vi "Topo & GridSpectr_DriftCorrection_zSpec_v19.vi"(6 "Internal use":string, 7 "Grid param":T1 {"height (m)" format="%#_6p"; "width (m)" format="%#_6p"; "center Y (m)" format="%#_6p"; "center X (m)" format="%#_6p"}, 8 "Error in (no error)":errorcluster, 9 "Points Y/Index Y":i32, 10 "Points X/Index X":i32, 11 "Method":enum16{"init", "run", "end"}(ring)=enum."end") -> (0 "Error out":errorcluster)   [LabVIEW 2014]
doc: "Example of a measurement VI to be used in the \"Experiments on a Grid\" tool as external VI.\n\nThis example measure the topography and spectroscopy data. The spectroscopy measurements are taken on a subgrid. The data are saved to a sxm and a binary file.\n\n- Nanonis Programming Interface -"
uses:
  <userlib>/Nanonis Prog Interface V5/Scan/Grid/GridPatternGet.vi
  <userlib>/Nanonis Prog Interface V5/Scan/Grid/LinePatternGet.vi
  <userlib>/Nanonis Prog Interface V5/Nanonis Prog Interface.lvlib
panel:
  in  "PLL ON/OFF":bool=TRUE
  in  "Spectroscopy":u16(ring) items=["Bias", "zSpec"]
  in  "autoStop":bool
  in  "trigger 2 >Hz":sgl format="%#_6p"
  in  "trigger1 < Hz":sgl format="%#_6p"
  out "zFile":refnum<file>
  out "last z adjustment":sgl=-8.2707174e-12 format="%#_6p"
  in  "during Spec Bias (V)":sgl=-0.1 format="%#_5p"
  in  "type":u16(ring)=1 items=["Line", "Grid"]
  in  "readjust setpoint every":i32=1
  in  "Correct Drift":bool=TRUE
  in  "Email when finished":string="cornelius.krull@monash.edu,Dhaneesh.Gopalakrishnan@monash.edu,marina.castelli@monash.edu"
  in  "STS z offset":dbl=2e-10 format="%#_6p"
  out "ETA":timestamp=timestamp(3575267058.899443 s since 1904-01-01)
  out "remaining":dbl format="%<%H:%M:%S>t"
  out "Progress":u8(slide)=100 scale=0.0..100.0 scale format="%#.1g"
  out "total Points":i32=2500
  in  "preSTS delay [ms]":u32=500
  in  "ref Bias":dbl=-0.1 format="%#_6p"
  in  "Imaging Bias":dbl=0.02 format="%#_6p"
  in  "max applied Drift Correction":i32=20 min=1 max=100 step=1 format="%.0p"
  in  "Correlate":u16(ring) items=["first Frame", "successive Frames"]
  out "Topo Images taken":i32=50
  in  "Increment":i32=8
  in  "Threshold":i32=2 min=1 step=1
  in  "tip Speed (m/s)":sgl=2e-09 format="%.2p"
  out "X drift":i32=1
  out "Y drift":i32
  out "Last Drift detected":i32=1
  in  "MaxImagesBack":i32=2
  in  "Channel index (0-23)":u8(ring) items=["Current"=0, "Z (m)"=14]
  in  "File name":string="symmetric_node_zOff=200p"
  in  "ref Current":dbl=7e-11 format="%#_6p"
  in  "Imaging Current":dbl=1e-11 format="%#_6p"
  in  "zdrift \nDuration (s)":dbl
  in  "Correct z drift":bool
  out "Status":string="finishing"
  in  "Drift correction Pixels":i32=256 caption="Topo Pixels"
  out "Y Offset":dbl=-4.101562475072873e-10 format="%#_6p"
  out "X Offset":dbl=4.687499971511855e-10 format="%#_6p"
  out "Points taken":dbl=2500.0
  in  "Drift Correction every":i32=80
  # "z Spectroscopy"
  # "GRID points"
  # "Increase this if no Drift was detected for \na certain number of images"
  # "%"
  # "time (HH:MM:SS)"
  # "images back"
  # "% of image size"
  # "RUN smart tilt before starting the GRID\nImg Angle = 0  CHECK CUTOFF\nmove tip to reference point for tip height"
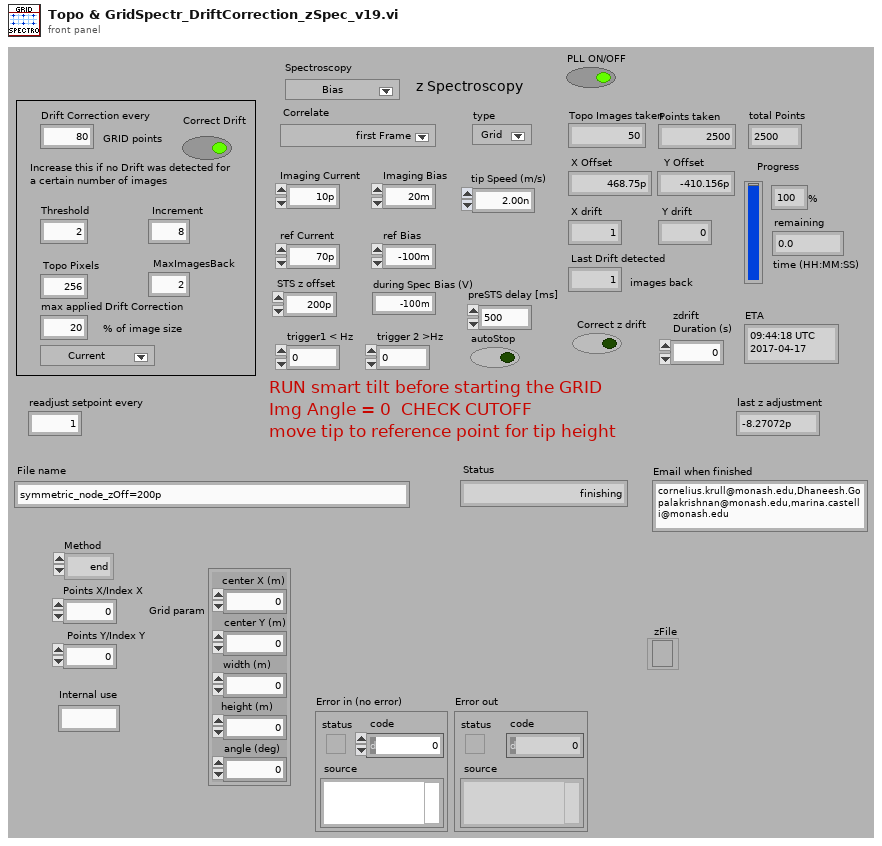
[diagram p1: front panel]
types:
  T1 = cluster{"center X (m)":sgl, "center Y (m)":sgl, "width (m)":sgl, "height (m)":sgl, "angle (deg)":sgl}
  T2 = enum16{"open", "replace", "create", "open or create", "replace or create", "replace or create with confirmation"}
  T3 = cluster{"Drift correction Pixels":i32, "Imaging Current":dbl, "STS Current":dbl, "MaxImagesBack":i32, "tip Speed (m/s)":sgl, "Threshold":i32, "Increment":i32, "Correlate":u16, "max applied Drift Correction":i32, "Imaging Bias":dbl, "Move Current":dbl, "Move Bias":dbl, "STS Bias":dbl, "preSTS delay [ms]":u32, "STS z offset":dbl, "Correct Drift":bool, "Lockin ON/OFF":bool}
  T4 = cluster{"x(m)":sgl, "y(m)":sgl, "Text":string, "Color":u32}
  T5 = cluster{"Z averaging time (s)":sgl, "Z offset (m)":sgl, "Initial settling time (s)":sgl}
  T6 = cluster{"center X":sgl, "center Y":sgl, "angle":sgl, "width":sgl, "height":sgl, "# pixels":i32, "# lines":i32}
  T7 = cluster{"Name":string, "Calibration":sgl, "Offset":sgl, "Channel index":i32}[]
  T8 = cluster{"up/down":bool, "time/line":sgl, "start time":timestamp, "end time":timestamp}
  T9 = cluster{"X (m)":sgl, "Y (m)":sgl, "Text":string, "Color":u32, "Visible":bool}[]
  T10 = cluster{"Max. slew rate (V/s)":sgl, "Settling time (s)":sgl, "Integration time (s)":sgl}
  T11 = cluster{"End settling time (s)":sgl, "Z control time (s)":sgl}
  T12 = cluster{"Z averaging time (s)":sgl, "Initial settling time (s)":sgl}
  T13 = cluster{"Max. slew rate (m/s)":sgl, "Settling time (s)":sgl, "Integration time (s)":sgl}
  T14 = cluster{"Points X/Index X":i32, "Points Y/Index Y":i32}
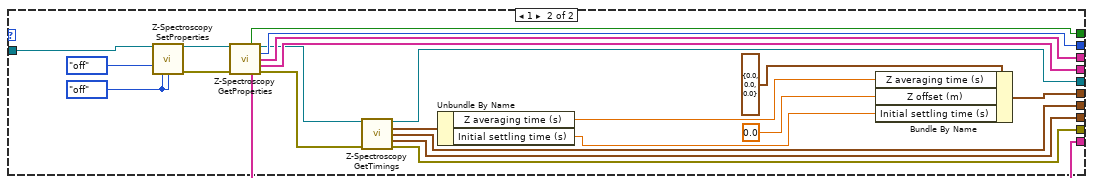
[diagram p3: hidden frame]
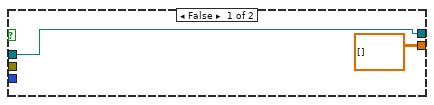
[diagram p4: hidden frame]
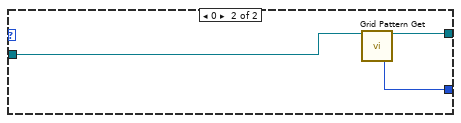
[diagram p5: hidden frame]
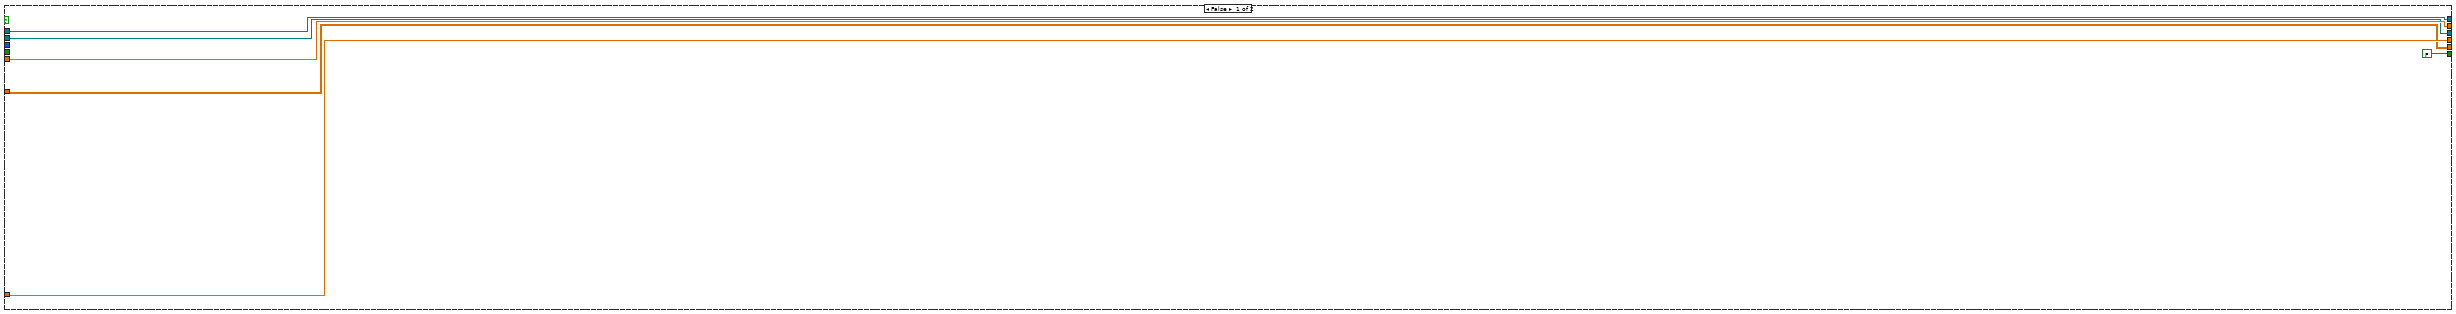
[diagram p10: hidden frame]
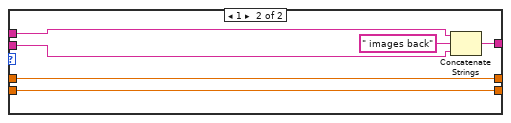
[diagram p11: hidden frame]
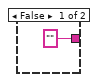
[diagram p13: hidden frame]
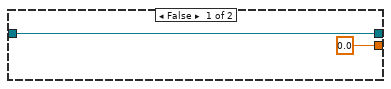
[diagram p14: hidden frame]
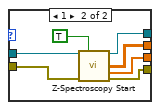
[diagram p16: hidden frame]
diagram:
  n1 = while {
    shift-right: [w21] -> _
    shift-left: _ -> [w38]
    shift-right: [w33] -> _
    shift-left: _ -> [w32]
    shift-right: [w30] -> _
    shift-left: _ -> [w31]
    shift-right: [w29] -> _
    shift-left: _ -> [w28]
    shift-right: [w27] -> _
    shift-left: _ -> [w26]
    shift-right: [w25] -> _
    shift-left: _ -> [w24]
    shift-right: [w23] -> _
    shift-left: _ -> [w22]
    shift-right: [w20] -> _
    shift-left: _ -> [w19]
    shift-right: [w18] -> _
    shift-left: _ -> [w17]
    shift-right: [w16] -> _
    shift-left: _ -> [w9]
    shift-right: [w15] -> _
    shift-left: _ -> [w8]
    shift-right: [w14] -> _
    shift-left: _ -> [w11]
    shift-right: [w13] -> _
    shift-left: _ -> [w10]
    shift-right: [w6] -> _
    shift-left: _ -> [w5]
    stop <- TRUE stop-if-true
    n2 = case shown="\"run\"" "Method" {
      tunnel: [w63 w296 _] -> w21
      tunnel: w38 -> [_ w296 w533]
      tunnel: "Error in (no error)" -> [w136 w289 w561]
      tunnel: [w118 w295 w501] -> w36
      tunnel: "Points X/Index X" -> [w56 w290 _]
      tunnel: "Points Y/Index Y" -> [w55 w283 _]
      tunnel: [w162 w293 w550] -> w33
      tunnel: w32 -> [_ w294 w550]
      tunnel: w31 -> [_ w292 w543]
      tunnel: [w154 w291 _] -> w30
      tunnel: [w152 w233 w573] -> w29
      tunnel: w28 -> [_ w233 w573]
      tunnel: [w108 w276 w512] -> w27
      tunnel: w26 -> [_ w260 w537]
      tunnel: ["Grid param" w286 _] -> w25
      tunnel: w24 -> [_ w286 w560]
      tunnel: [w134 w251 _] -> w23
      tunnel: w22 -> [_ w251 w568]
      tunnel: [w55 w284 w551] -> w20
      tunnel: w19 -> [_ w284 w551]
      tunnel: [w56 w285 w552] -> w18
      tunnel: w17 -> [_ w285 w552]
      tunnel: [w145 w266 w549] -> w16
      tunnel: [w145 w271 w547] -> w15
      tunnel: [w130 w265 w544] -> w14
      tunnel: [0 w249 w548] -> w13
      tunnel: w10 -> [_ w235 w548]
      tunnel: "Drift Correction every" -> [_ w279 _]
      tunnel: w11 -> [_ w270 w544]
      tunnel: w9 -> [_ w277 w549]
      tunnel: w8 -> [_ w263 w547]
      tunnel: "Drift correction Pixels" -> [w129 _ _]
      tunnel: [w105 w268 _] -> w6
      tunnel: w5 -> [_ w269 w545]
      tunnel: "Correct z drift" -> [_ w267 _]
      tunnel: "Channel index (0-23)" -> [w87 w264 _]
      tunnel: "MaxImagesBack" -> [w128 _ _]
      tunnel: "Correlate" -> [w114 _ _]
      frame "init", Default {
        w65 = 0.0 ("Move Current")
        w145 = 0.0
        # "- Get bias spectroscopy parameters\n- Open binary file for spectr. data"
        # "initialize Z buffer"
        # "Get index of Z in Signal list"
        n3 = case shown="0, Default" w114 {
          frame 0, Default {
            n4 = local write "MaxImagesBack"(2 ("StepsBack")) -> ()
          }
          frame 1 {
          }
        }
        n5 = call <userlib>:"Prog Interface - OpenAppRef.vi"("Error in (no error)"=w136) -> ("Error out"=w83:errorcluster, "Application reference"=w84:refnum<vi>)  [unwired: 5 in]
        n6 = local write "Status"("init" ("Status")) -> ()
        n7 = call <userlib>:"XY-Pos Get.vi"("error in (no error)"=w83, "Application ref in"=w84) -> ("error out"=w52:errorcluster, "Y (m)"=w77:sgl, "X (m)"=w78:sgl, "Application ref out"=w48:refnum<vi>)  [unwired: 5 in]
        n8 = call <userlib>:"Points Get.vi"("Application ref in"=w48) -> ("Application ref out"=w47:refnum<vi>, "Points"=w49:T9)  [unwired: 12 in, 1 out]
        n9 = for {
          tunnel: w49 -> [w169] mode=indexing
          tunnel: [w163] -> w44 mode=indexing
          n10 = Unbundle By Name(w169) -> ("X (m)"=w167:sgl, "Y (m)"=w166:sgl, "Text"=w165:string, "Color"=w164:u32)  [unwired: 1 out]
          n11 = Bundle By Name(cluster=T4 {"x(m)"=0.0, "y(m)"=0.0, "Text"="", "Color"=16777216} ("Point"), "x(m)"=w167, "y(m)"=w166, "Text"=w165, "Color"=w164) -> (w163:T4)
        }
        n12 = Bundle By Name(cluster=cluster{"X (m)":sgl, "Y (m)":sgl} {"X (m)"=0.0, "Y (m)"=0.0} ("Point Coordinates"), "X (m)"=w78, "Y (m)"=w77) -> (w79:cluster{"X (m)":sgl, "Y (m)":sgl})
        n13 = call <userlib>:"Point Erase.vi"("Application ref in"=w47, "Point index (-1=All points)"=-1) -> ("Application ref out"=w70:refnum<vi>)  [unwired: 12 in, 1 out]
        n14 = call <userlib>:"Point Draw.vi"("Application ref in"=w70, "Point Coordinates"=w79, "Text"="ref X ref", "Color"=u32 6618880) -> ("Application ref out"=w46:refnum<vi>)  [unwired: 10 in, 1 out]
        n15 = call <userlib>:"Points Draw.vi"("Application ref in"=w46, "Points Configuration"=w44) -> ("Application ref out"=w45:refnum<vi>)  [unwired: 12 in, 1 out]
        n16 = call <userlib>:"Point ShowHide.vi"("Application ref in"=w45, "Point index (-1=All points)"=-1, "Show/Hide"=enum16{"Show", "Hide"}."Show") -> ("Application ref out"=w73:refnum<vi>)  [unwired: 11 in, 1 out]
        n17 = case shown="1, Default" "type" {
          tunnel: [w223 w226] -> w51
          tunnel: [w220 w224] -> w109
          tunnel: w73 -> [w219 w225]
          frame 1, Default {
            n18 = call-poly <userlib>:"Grid Pattern Get.vi"("Application ref in"=w219) -> ("Points Y"=w221:i32, "Points X"=w222:i32, "Application ref out"=w223:refnum<vi>)  [unwired: 10 in, 6 out]
            n19 = Multiply(x=w221, y=w222) -> (x*y=w220:i32)
          }
          frame 0 {
            n20 = call-poly <userlib>:"Grid Pattern Get.vi"("Application ref in"=w225) -> ("Points"=w224:i32, "Application ref out"=w226:refnum<vi>)  [unwired: 12 in, 5 out]
          }
        }
        "total Points" <- w109
        n21 = local write "Topo Images taken"(0 ("Images taken")) -> ()
        n22 = local write "Last Drift detected"(0 ("Last Drift detected")) -> ()
        n23 = call <userlib>:"Get Session Path.vi"("error in (no error)"=w52, "Application ref in"=w51) -> ("error out"=w135:errorcluster, "Session path"=w122:path, "Application ref out"=w116:refnum<vi>)  [unwired: 7 in]
        n24 = local read "Spectroscopy"() -> (w53:u16)
        n25 = Get Date/Time In Seconds() -> (seconds since 1Jan1904=w134:timestamp)
        n26 = case shown="0, Default" w53 {
          tunnel: [w171 w206] -> w158
          tunnel: [w174 w205] -> w156
          tunnel: [w178 w192] -> w155
          tunnel: [w173 w204] -> w151
          tunnel: [w172 w203] -> w149
          tunnel: [w175 w202] -> w148
          tunnel: w116 -> [w180 w195]
          tunnel: [w177 w200] -> w76
          tunnel: [w176 w199] -> w75
          tunnel: [w170 w185] -> w50
          tunnel: [w179 w198] -> w54
          frame 0, Default {
            n27 = call <userlib>:"BiasSpectroscopy SetProperties.vi"("Application ref in"=w180) -> ("Application ref out"=w184:refnum<vi>, "Error out"=w183:errorcluster)  [unwired: 13 in]
            n28 = call <userlib>:"BiasSpectroscopy GetProperties.vi"("Application ref in"=w184, "Error in (no error)"=w183) -> ("Backward sweep"=w171:bool, "Application ref out"=w182:refnum<vi>, "Number of points"=w172:i32, "Channels"=w175:string[], "Parameters"=w174:string[], "Fixed parameters"=w173:string[], "Error out"=w181:errorcluster)  [unwired: 5 in, 2 out]
            n29 = call <userlib>:"BiasSpectroscopy GetTimings.vi"("Application ref in"=w182, "Error in (no error)"=w181) -> ("Application ref out"=w179:refnum<vi>, "Initialization"=w170:T5, "Sweep Timing"=w176:T10, "End of Sweep"=w177:T11, "Error out"=w178:errorcluster)  [unwired: 9 in]
          }
          frame 1 {
            w197 = enum16{"no change", "on", "off"}."off" ("Save dialog")
            n30 = call <userlib>:"Z-Spectroscopy SetProperties.vi"("Application ref in"=w195, "Autosave"=enum16{"no change", "on", "off"}."off" ("Autosave (no change)"), "Save dialog"=w197, "Save all sweeps (no change)"=w197) -> ("Application ref out"=w194:refnum<vi>, "error out"=w193:errorcluster)  [unwired: 10 in]
            n31 = call <userlib>:"Z-Spectroscopy GetProperties.vi"("Application ref in"=w194, "error in (no error)"=w193) -> ("Backward sweep"=w206:bool, "Application ref out"=w201:refnum<vi>, "Number of points"=w203:i32, "Channels"=w202:string[], "Parameters"=w205:string[], "Fixed parameters"=w204:string[], "error out"=w191:errorcluster)  [unwired: 6 in, 1 out]
            n32 = call <userlib>:"Z-Spectroscopy GetTimings.vi"("Application ref in"=w201, "Error in (no error)"=w191) -> ("Application ref out"=w198:refnum<vi>, "Initialization"=w186:T12, "Sweep Timing"=w199:T13, "End of Sweep"=w200:T11, "Error out"=w192:errorcluster)  [unwired: 9 in]
            n33 = Unbundle By Name(w186) -> ("Z averaging time (s)"=w188:sgl, "Initial settling time (s)"=w189:sgl)
            n34 = Bundle By Name(cluster=T5 {"Z averaging time (s)"=0.0, "Z offset (m)"=0.0, "Initial settling time (s)"=0.0} ("Initialization"), "Z averaging time (s)"=w188, "Z offset (m)"=sgl 0.0, "Initial settling time (s)"=w189) -> (w185:T5)
          }
        }
        n35 = call "Create Filenames (SubVI).vi"("error in (no error)"=w135, "seconds since 1Jan1904"=w134, "File name"="File name", "Session path"=w122) -> ("error out"=w125:errorcluster, "binFilePath"=w119:path, "topoFilePath"=w63:path, "Drift File out"=w106:refnum<file>)  [unwired: 4 in]
        n36 = Strip Path(path=w63) -> (stripped path=w62:path)  [unwired: 1 out]
        n37 = Strip Path(path=w119) -> (stripped path=w121:path)  [unwired: 1 out]
        n38 = Build Path(base path=w121, name or relative path="topo") -> (appended path=w43:path)
        n39 = Build Path(base path=w62, name or relative path="zAdjustments.txt") -> (appended path=w60:path)
        n40 = Open/Create/Replace File(file path (use dialog)=w60, operation (0:open)=T2."open or create", access (0:read/write)=enum16{"read/write", "read-only", "write-only"}."write-only") -> (refnum out=→"zFile":refnum<file>)  [unwired: 3 in, 2 out]
        n41 = local read "max applied Drift Correction"() -> (w93:i32)
        n42 = local read "Drift correction Pixels"() -> (w101:i32)
        n43 = local read "preSTS delay [ms]"() -> (w90:u32)
        n44 = local read "Imaging Current"() -> (w100:dbl)
        n45 = local read "MaxImagesBack"() -> (w97:i32)
        n46 = local read "tip Speed (m/s)"() -> (w98:sgl)
        n47 = local read "Imaging Bias"() -> (w92:dbl)
        n48 = local read "Correct Drift"() -> (w88:bool)
        n49 = local read "STS z offset"() -> (w89:dbl)
        n50 = local read "ref Current"() -> (w99:dbl)
        n51 = local read "Increment"() -> (w95:i32)
        n52 = local read "Threshold"() -> (w96:i32)
        n53 = local read "Correlate"() -> (w94:u16)
        n54 = local read "ref Bias"() -> (w91:dbl)
        n55 = Bundle By Name(cluster=T3 {"Drift correction Pixels"=256, "Imaging Current"=5e-11, "STS Current"=1e-10, "MaxImagesBack"=2, "tip Speed (m/s)"=1e-08, "Threshold"=2, "Increment"=64, "Correlate"=0, "max applied Drift Correction"=20, "Imaging Bias"=-0.02, "Move Current"=1.5e-11, "Move Bias"=-0.02, "STS Bias"=0.1, "preSTS delay [ms]"=1000, "STS z offset"=-1.7e-10, "Correct Drift"=TRUE, "Lockin ON/OFF"=TRUE} ("Drift Correction"), "Drift correction Pixels"=w101, "Imaging Current"=w100, "STS Current"=w99, "MaxImagesBack"=w97, "tip Speed (m/s)"=w98, "Threshold"=w96, "Increment"=w95, "Correlate"=w94, "max applied Drift Correction"=w93, "Imaging Bias"=w92, "Move Current"=w65, "Move Bias"=w65, "STS Bias"=w91, "preSTS delay [ms]"=w90, "STS z offset"=w89, "Correct Drift"=w88, "Lockin ON/OFF"=FALSE) -> (w103:T3)
        n56 = Bundle("Points X/Index X"=w56, "Points Y/Index Y"=w55) -> (w157:T14)  [unwired: 1 in]
        n57 = call "DriftFileHeader(SubVI).vi"("Byte Stream File in"=w106, "Drift Correction"=w103, "End of Sweep"=w76, "Application ref in"=w54, "Sweep Timing"=w75, "Initialization"=w50) -> ("Byte Stream File out"=w105:refnum<file>, "Application ref out"=w104:refnum<vi>)  [unwired: 8 in]
        n58 = call <userlib>:"Create Header for BinaryFile.vi"("Grid points"=w157, "Grid param"="Grid param", "Fixed parameters"=w151, "Backward sweep"=w158, "Sweep signal"="Bias (V)" ("Sweep Signal"), "Parameters"=w156, "Channels"=w148, "Points per sweep"=w149) -> ("Header (fixed attributes)"=w160:string[][])  [unwired: 3 in]
        n59 = call <userlib>:"Write Header to BinaryFile [ with Save dialog].vi"("Fixed Attributes"=w160, "Show Dialog? (T)"=FALSE, "Filename"=w119) -> ("Error out"=w126:errorcluster, "File ref"=w154:refnum<file>)  [unwired: 5 in, 2 out]
        n60 = local read "Imaging Bias"() -> (w111:dbl)
        n61 = Merge Errors(w126, w125) -> (w127:errorcluster)
        n62 = call "SafeBiasSet.vi"("Application ref in"=w104, "Bias (V)"=w111) -> ("Application ref out"=w42:refnum<vi>)  [unwired: 7 in, 1 out]
        n63 = Merge Errors(w155, w127) -> (w118:errorcluster)
        n64 = call <userlib>:"Set Session Path.vi"("error in (no error)"=w118, "Session Folder"=w43, "Application ref in"=w42) -> ("error out"=w117:errorcluster, "Application ref out"=w41:refnum<vi>)  [unwired: 7 in]
        n65 = local read "Imaging Current"() -> (w110:dbl)
        n66 = call <userlib>:"Z-Ctrl Setpoint Set.vi"("error in (no error)"=w117, "Z Controller setpoint"=w110, "Application ref in"=w41) -> ("error out"=w137:errorcluster, "Application ref out"=w138:refnum<vi>)  [unwired: 7 in]
        n67 = call <userlib>:"Signal Names Get.vi"("error in (no error)"=w137, "Application ref in"=w138) -> ("error out"=w86:errorcluster, "Signals Names"=w150:string[], "Application ref out"=w141:refnum<vi>)  [unwired: 5 in]
        n68 = Search 1D Array(1D array=w150, element="Z (m)") -> (index of element=w152:i32)  [unwired: 1 in]
        n69 = call <userlib>:"Scan SetProperties.vi"("Application ref in"=w141, "Continuous scan"=enum16{"No change", "On", "Off"}."Off") -> ("Application ref out"=w143:refnum<vi>, "Error out"=w142:errorcluster)  [unwired: 12 in]
        n70 = call <userlib>:"ScanBuffer Set.vi"("Application ref in"=w143, "Pixels"=w129, "Lines"=w129, "error in (no error)"=w142) -> ("Application ref out"=w112:refnum<vi>)  [unwired: 10 in, 1 out]
        n71 = call <userlib>:"FolMe Speed Set.vi"("Speed Setting (Custom)"=enum32{"Scan speed", "Custom speed"}."Custom speed", "Speed (m/s)"="tip Speed (m/s)", "Application ref in"=w112) -> ("Application ref out"=w68:refnum<vi>)  [unwired: 5 in, 1 out]
        n72 = local read "Correct Drift"() -> (w66:bool)
        n73 = case shown="True" w66 {
          tunnel: w87 -> [_ w218]
          tunnel: w86 -> [_ w217]
          tunnel: [dbl[][] [] ("Array") w216] -> w85
          tunnel: w68 -> [w208 w214]
          tunnel: [w208 w210] -> w64
          frame False {
          }
          frame True {
            n74 = call "PLL_On_Off (SubVI).vi"("Output ON/OFF (F=OFF)"=FALSE, "Application in"=w214) -> ("Application out"=w213:refnum<vi>)  [unwired: 8 in, 1 out]
            n75 = local read "PLL ON/OFF"() -> (w209:bool)
            n76 = call "Scan_normailze(SubVI).vi"("error in (no error)"=w217, "Channel index (0-23)"=w218, "Normalization"=FALSE ("Boolean"), "Application in"=w213) -> ("Array"=w216:dbl[][], "Application out"=w211:refnum<vi>)  [unwired: 5 in, 1 out]
            n77 = call "PLL_On_Off (SubVI).vi"("Output ON/OFF (F=OFF)"=w209, "Application in"=w211) -> ("Application out"=w210:refnum<vi>)  [unwired: 8 in, 1 out]
          }
        }
        n78 = Initialize Array(0.0 ("element"), w128, w129, w129) -> (w131:dbl[][][])
        n79 = for {
          N: w128 -> [_]
          tunnel: w85 -> [w230]
          shift-right: [w229] -> w130
          shift-left: w131 -> [w231]
          i -> [w228]
          n80 = Replace Array Subset(array=w231, new element=w230, index (dim 0)=w228) -> (w229:dbl[][][])  [unwired: 2 in]
        }
        n81 = call <userlib>:"BiasSpectroscopy SetProperties.vi"("Application ref in"=w64, "Z-Controller hold (no change)"=enum16{"no change", "on", "off"}."off") -> ("Application ref out"=w108:refnum<vi>)  [unwired: 12 in, 1 out]
        n82 = Initialize Array(sgl nan ("element"), w55, w56) -> (w162:sgl[][])
      }
      frame "run" {
        # "shift tip position"
        # "Get Z position"
        # "- get Z position for topography and store it to Z buffer\n- if x,y indices are a multiple of the spacings, take spectroscopy curve and write data to binary file\ndo drift correction if number of STS position was reached"
        n83 = Quotient & Remainder(x=w235, y=w279) -> (x-y*floor(x/y)=w280:i32)  [unwired: 1 out]
        n84 = Equal To 0?(x=w280) -> (x = 0?=w278:bool)
        n85 = Not Equal To 0?(x=w235) -> (x != 0?=w261:bool)
        n86 = local read "Correct Drift"() -> (w243:bool)
        n87 = Compound Arithmetic op=AND(w261, w278, w243) -> (w262:bool)
        n88 = call <userlib>:"XY-Pos Get.vi"("Wait for newest data (F=False)"=TRUE, "Application ref in"=w260) -> ("Y (m)"=w256:sgl, "X (m)"=w257:sgl, "Application ref out"=w259:refnum<vi>)  [unwired: 5 in, 1 out]
        n89 = case shown="True" w262 {
          tunnel: w259 -> [w357 w369]
          tunnel: [w357 w414] -> w240
          tunnel: w270 -> [w354 w410]
          tunnel: [w356 w412] -> w266
          tunnel: [w355 w411] -> w271
          tunnel: w277 -> [w356 w393]
          tunnel: w263 -> [w355 w391]
          tunnel: [w354 w406] -> w265
          tunnel: w269 -> [w353 w417]
          tunnel: [w353 w416] -> w268
          tunnel: w267 -> [_ w413]
          tunnel: w264 -> [_ w397]
          tunnel: [FALSE TRUE] -> w237
          frame False {
          }
          frame True {
            # "Drift correction \ncompare to the reference image with the previous image \ndx and dy will be applied to the grid coord, \nand the imaging frame will be shifted"
            n90 = Greater Or Equal To 0?(x=w397) -> (x >= 0?=w396:bool)
            n91 = case shown="True" w396 {
              frame False {
              }
              frame True {
                n92 = local read "Topo Images taken"() -> (w432:i32)
                n93 = Increment(x=w432) -> (x+1=w431:i32)
                n94 = local write "Topo Images taken"(w431) -> ()
              }
            }
            n95 = local read "Imaging Bias"() -> (w376:dbl)
            n96 = call "move2mark (SubVI).vi"("Application in"=w369) -> ("Application out"=w368:refnum<vi>)  [unwired: 10 in]
            n97 = local read "Imaging Current"() -> (w375:dbl)
            n98 = local write "Status"("Drift Correction" ("Status")) -> ()
            n99 = call "SafeBiasSet.vi"("Application ref in"=w368, "Bias (V)"=w376) -> ("Application ref out"=w377:refnum<vi>)  [unwired: 7 in, 1 out]
            n100 = call <userlib>:"Z-Ctrl Setpoint Set.vi"("Z Controller setpoint"=w375, "Application ref in"=w377) -> ("Application ref out"=w367:refnum<vi>)  [unwired: 8 in, 1 out]
            n101 = call <userlib>:"Ctrl-on_off Set.vi"("Z Controller ON/OFF"=TRUE, "Application ref in"=w367) -> ("Application ref out"=w365:refnum<vi>)  [unwired: 8 in, 1 out]
            n102 = call "PLL_On_Off (SubVI).vi"("Output ON/OFF (F=OFF)"=FALSE, "Application in"=w365) -> ("Application out"=w364:refnum<vi>)  [unwired: 8 in, 1 out]
            n103 = local read "Drift correction Pixels"() -> (w385:i32)
            n104 = local read "Last Drift detected"() -> (w388:i32)
            n105 = call "Scan_normailze(SubVI).vi"("Channel index (0-23)"=w397, "Normalization"=FALSE ("Boolean"), "Application in"=w364) -> ("Array"=w407:dbl[][], "Application out"=w362:refnum<vi>)  [unwired: 6 in, 1 out]
            n106 = local read "Correlate"() -> (w394:u16)
            n107 = Divide(x="max applied Drift Correction", y=100) -> (x/y=w384:dbl)
            n108 = Multiply(x=w384, y=w385) -> (x*y=w386:dbl)
            n109 = call "PLL_On_Off (SubVI).vi"("Output ON/OFF (F=OFF)"="PLL ON/OFF", "Application in"=w362) -> ("Application out"=w360:refnum<vi>)  [unwired: 8 in, 1 out]
            n110 = call "CorrelImages (SubVI)v2.vi"("last drift detected"=w388, "Correlate"=w394, "Ref Array"=w410, "New Image"=w407) -> ("Y drift"=w382:i32, "X drift"=w379:i32, "Ref Array out"=w406:dbl[][][], "Queue Steps"=w395:i32)  [unwired: 4 in]
            "X drift" <- w379
            "Y drift" <- w382
            "Last Drift detected" <- w395
            n111 = local read "Topo Images taken"() -> (w399:i32)
            n112 = To Long Integer(number=w386) -> (32bit integer=w378:i32)
            n113 = Greater Or Equal?(x=w395, y="Threshold") -> (x >= y?=w401:bool)
            n114 = Greater?(x=w399, y="Threshold") -> (0:w398:bool)
            n115 = call "AbsLimit (SubVI).vi"("in"=w379, "Abslimt"=w378) -> ("Numeric out"=w381:i32)  [unwired: 9 in]
            n116 = call "AbsLimit (SubVI).vi"("in"=w382, "Abslimt"=w378) -> ("Numeric out"=w380:i32)  [unwired: 9 in]
            n117 = And(x=w401, y=w398) -> (x .and. y?=w400:bool)
            n118 = case shown="True" w400 {
              tunnel: ["" w436] -> w402
              frame False {
              }
              frame True {
                n119 = local write "Last Drift detected"(0 ("Last Drift detected")) -> ()
                n120 = local read "Drift Correction every"() -> (w435:i32)
                n121 = Add(x=w435, y="Increment") -> (x+y=w439:i32)
                n122 = local write "Drift Correction every"(w439) -> ()
                n123 = Number To Decimal String(number=w439) -> (decimal integer string=w438:string)  [unwired: 1 in]
                n124 = Concatenate Strings(" Increased DC to every " ("string"), w438) -> (w436:string)
              }
            }
            n125 = local read "Drift correction Pixels"() -> (w404:i32)
            n126 = call "drift_pixel2m (SubVI).vi"("Application in"=w360, "X drift"=w381, "Y drift"=w380, "Drift correction Pixels"=w404) -> ("Application out"=w403:refnum<vi>, "x drift"=w373:sgl, "y drift"=w372:sgl)  [unwired: 2 in, 1 out]
            n127 = call "ShiftFrame (SubVI).vi"("Y shift"=w372, "X shift"=w373, "Application in"=w403) -> ("Application out"=w405:refnum<vi>)  [unwired: 8 in]
            n128 = local read "type"() -> (w359:u16)
            n129 = call "MoveGrid.vi"("type"=w359, "y"=w372, "x"=w373, "Application ref in"=w405) -> ("Application ref out"=w371:refnum<vi>)  [unwired: 6 in, 1 out]
            n130 = call "shift marks (SubVI).vi"("y"=w372, "x"=w373, "Application in"=w371) -> ("Application out"=w370:refnum<vi>)  [unwired: 7 in, 1 out]
            n131 = case shown="True" w413 {
              tunnel: [0.0 ("z drift") w446] -> w415
              tunnel: w370 -> [w441 w445]
              tunnel: [w441 w444] -> w414
              frame False {
              }
              frame True {
                n132 = call "Zdrift_subVi.vi"("Duration"="zdrift \nDuration (s)", "Application in"=w445) -> ("z drift"=w446:dbl, "Application out"=w444:refnum<vi>)  [unwired: 7 in, 1 out]
              }
            }
            n133 = Number To Decimal String(number=w395) -> (decimal integer string=w409:string)  [unwired: 1 in]
            n134 = case shown="0, Default" w394 {
              tunnel: w409 -> [w419 w430]
              tunnel: [w424 w429] -> w408
              tunnel: w402 -> [w422 w427]
              tunnel: w393 -> [w420 w426]
              tunnel: [w420 w426] -> w392
              tunnel: w391 -> [w421 w425]
              tunnel: [w421 w425] -> w390
              frame 0, Default {
                n135 = Concatenate Strings(w419, "images back , Correlating first frame " ("string"), w422) -> (w424:string)
              }
              frame 1 {
                n136 = Concatenate Strings(w430, " images back" ("string"), w427) -> (w429:string)
              }
            }
            n137 = Add(x=w392, y=w373) -> (x+y=w412:dbl)
            n138 = Add(x=w372, y=w390) -> (x+y=w411:dbl)
            n139 = local write "X Offset"(w412) -> ()
            n140 = call "Drift Data to file (SubVI).vi"("z drift"=w415, "Comment"=w408, "y Drift"=w411, "X drift"=w412, "Byte Stream File in"=w417) -> ("Byte Stream File out"=w416:refnum<file>)  [unwired: 6 in]
            n141 = local write "Y Offset"(w411) -> ()
          }
        }
        n142 = Quotient & Remainder(x=w235, y="readjust setpoint every") -> (x-y*floor(x/y)=w236:i32)  [unwired: 1 out]
        n143 = Equal To 0?(x=w236) -> (x = 0?=w239:bool)
        n144 = Equal To 0?(x=w235) -> (x = 0?=w234:bool)
        n145 = Add(x=w257, y=w266) -> (x+y=w273:dbl)
        n146 = Add(x=w256, y=w271) -> (x+y=w272:dbl)
        n147 = Compound Arithmetic op=OR(w234, w237, w239) -> (w238:bool)
        n148 = case shown="True" w238 {
          tunnel: [w297 w314] -> w241
          tunnel: w240 -> [w297 w330]
          tunnel: w233 -> [_ w316]
          frame False {
          }
          frame True {
            n149 = call "move2mark (SubVI).vi"("Application in"=w330) -> ("Application out"=w319:refnum<vi>)  [unwired: 10 in]
            n150 = local read "ref Bias"() -> (w329:dbl)
            n151 = call <userlib>:"Signal Value Get (Animation period) v2.vi"("Wait for newest data (F=False)"=TRUE, "Signal index (0-79)"=w316, "Application ref in"=w319) -> ("Signal value"=w312:sgl, "Application ref out"=w318:refnum<vi>)  [unwired: 5 in, 1 out]
            n152 = local read "ref Current"() -> (w326:dbl)
            n153 = local write "Status"("adjust setpoint" ("Status")) -> ()
            n154 = call "SafeBiasSet.vi"("Application ref in"=w318, "Bias (V)"=w329) -> ("Application ref out"=w327:refnum<vi>)  [unwired: 7 in, 1 out]
            n155 = flat-sequence {
              tunnel: w327 -> [w335]
              tunnel: [w332] -> w325
              tunnel: w326 -> [w334]
              tunnel: w325 -> [w338]
              tunnel: [w338] -> w324
              tunnel: "preSTS delay [ms]" -> [w336]
              tunnel: w324 -> [w343]
              tunnel: [w340] -> w328
              tunnel: [w341] -> w322
              tunnel: w328 -> [w347]
              tunnel: "preSTS delay [ms]" -> [w346]
              tunnel: w322 -> [_]
              tunnel: [w347] -> w320
              tunnel: [w349] -> w315
              tunnel: w320 -> [w350]
              frame #0 {
                n156 = call <userlib>:"Z-Ctrl Setpoint Set.vi"("Z Controller setpoint"=w334, "Application ref in"=w335) -> ("Application ref out"=w333:refnum<vi>)  [unwired: 8 in, 1 out]
                n157 = call <userlib>:"Ctrl-on_off Set.vi"("Z Controller ON/OFF"=TRUE, "Application ref in"=w333) -> ("Application ref out"=w332:refnum<vi>)  [unwired: 8 in, 1 out]
              }
              frame #1 {
                n158 = Greater Than 0?(x=w336) -> (x > 0?=w337:bool)
                n159 = case shown="True" w337 {
                  tunnel: w336 -> [_ w339]
                  frame False {
                  }
                  frame True {
                    n160 = Wait (ms)(milliseconds to wait=w339) -> ()  [unwired: 1 out]
                  }
                }
              }
              frame #2 {
                n161 = local read "STS z offset"() -> (w341:dbl)
                n162 = call <userlib>:"TipLift Set.vi"("TipLift (m)"=w341, "Application ref in"=w343) -> ("Application ref out"=w342:refnum<vi>)  [unwired: 8 in, 1 out]
                n163 = call <userlib>:"Ctrl-on_off Set.vi"("Z Controller ON/OFF"=FALSE, "Application ref in"=w342) -> ("Application ref out"=w340:refnum<vi>)  [unwired: 8 in, 1 out]
              }
              frame #3 {
                n164 = Greater Than 0?(x=w346) -> (x > 0?=w345:bool)
                n165 = case shown="True" w345 {
                  tunnel: w346 -> [_ w348]
                  frame False {
                  }
                  frame True {
                    n166 = Wait (ms)(milliseconds to wait=w348) -> ()  [unwired: 1 out]
                  }
                }
              }
              frame #4 {
                n167 = call "SafeBiasSet.vi"("Application ref in"=w350, "Bias (V)"="during Spec Bias (V)") -> ("Application ref out"=w349:refnum<vi>)  [unwired: 7 in, 1 out]
              }
            }
            n168 = Get Date/Time In Seconds() -> (seconds since 1Jan1904=w303:timestamp)
            n169 = call <userlib>:"Signal Value Get (Animation period) v2.vi"("Wait for newest data (F=False)"=TRUE, "Signal index (0-79)"=w316, "Application ref in"=w315) -> ("Signal value"=w311:sgl, "Application ref out"=w314:refnum<vi>)  [unwired: 5 in, 1 out]
            n170 = Get Date/Time String(date format (0)=enum16{"short", "long", "abbreviated"}."short", seconds (now)=w303, want seconds? (F)=TRUE) -> (date string=w307:string, time string=w306:string)
            n171 = Subtract(x=w312, y=w311) -> (x-y=w309:sgl)
            "last z adjustment" <- w309
            n172 = Concatenate Strings(w307, w306, "," ("string")) -> (w305:string)
            n173 = Format Into String(format string="%#g", initial string=w305, w309) -> (resulting string=w300:string)  [unwired: 1 in, 1 out]
            n174 = Concatenate Strings(w300, "\r\n") -> (w299:string)
            n175 = local read "zFile"() -> (w310:refnum<file>)
            n176 = Write to Text File(file (use dialog)=w310, text=w299) -> ()  [unwired: 2 in, 3 out]
          }
        }
        n177 = Subtract(x=w284, y=w283) -> (x-y=w282:i32)
        n178 = call <userlib>:"XY-Pos Set.vi"("Y (m)"=w272, "X (m)"=w273, "Application ref in"=w241) -> ("Application ref out"=w274:refnum<vi>)  [unwired: 5 in, 1 out]
        n179 = Decrement(x=w282) -> (x-1=w281:i32)
        n180 = call <userlib>:"Signal Value Get (Animation period).vi"("error in (no error)"=w289, "Signal index (0-47)"=w233, "Application ref in"=w274) -> ("error out"=w288:errorcluster, "Signal value"=w287:sgl, "Application ref out"=w275:refnum<vi>)  [unwired: 5 in]
        n181 = Replace Array Subset(array=w294, new element=w287, index (row)=w281, index (col)=w290) -> (w293:sgl[][])
        n182 = case shown="True" TRUE {
          tunnel: [w449 w453] -> w295
          tunnel: w292 -> [w450 w473]
          tunnel: [w450 w471] -> w291
          tunnel: w288 -> [w449 w456]
          tunnel: w275 -> [w448 w457]
          tunnel: [w448 w458] -> w276
          tunnel: [w447 w460] -> w249
          tunnel: w235 -> [w447 w461]
          frame False {
            # "Point indices aren't multiple of subgrid spacing\n=> no spectroscopy at this point"
          }
          frame True {
            n183 = local write "Status"("zSpec" ("Status")) -> ()
            n184 = case shown="True" "autoStop" {
              tunnel: w457 -> [_ w493]
              tunnel: w456 -> [w488 w490]
              tunnel: [w488 w489] -> w455
              frame False {
              }
              frame True {
                n185 = call "zSpec_trigger.vi"("Error in (no error)"=w490, "trigger 2"="trigger 2 >Hz", "trigger1"="trigger1 < Hz", "Application ref in"=w493) -> ("Error out"=w489:errorcluster)  [unwired: 5 in, 1 out]
              }
            }
            n186 = case shown="0, Default" "Spectroscopy" {
              tunnel: [w474 w487] -> w470
              tunnel: [w475 w486] -> w469
              tunnel: [w476 w484] -> w463
              tunnel: [w477 w483] -> w458
              tunnel: w457 -> [w479 w482]
              tunnel: w456 -> [w478 w481]
              frame 0, Default {
                n187 = call <userlib>:"BiasSpectroscopy Start.vi"("Application ref in"=w479, "Get data (F)"=TRUE, "Error in (no error)"=w478) -> ("Application ref out"=w477:refnum<vi>, "Data"=w474:sgl[][], "Parameters"=w475:sgl[], "Error out"=w476:errorcluster)  [unwired: 8 in, 1 out]
              }
              frame 1 {
                n188 = call <userlib>:"Z-Spectroscopy Start.vi"("Application ref in"=w482, "Get data (F=False)"=TRUE ("Get Data (F)"), "error in (no error)"=w481) -> ("Application ref out"=w483:refnum<vi>, "Data"=w487:sgl[][], "Parameters"=w486:sgl[], "error out"=w484:errorcluster)  [unwired: 8 in, 1 out]
              }
            }
            n189 = Delete From Array(array=w470, length=1, index (row)=0 ("index")) -> (array with subset deleted=w468:sgl[][])  [unwired: 1 in, 1 out]
            n190 = Write to Binary File(file (use dialog)=w473, data=w469, error in=w463, 5:FALSE ("prepend array or string size? (T)")) -> (refnum out=w472:refnum<file>, error out=w462:errorcluster)  [unwired: 2 in, 1 out]
            n191 = Write to Binary File(file (use dialog)=w472, data=w468, error in=w462, 5:FALSE ("prepend array or string size? (T)")) -> (refnum out=w471:refnum<file>, error out=w454:errorcluster)  [unwired: 2 in, 1 out]
            n192 = Increment(x=w461) -> (x+1=w460:i32)
            n193 = Merge Errors(w455, w454) -> (w453:errorcluster)
          }
        }
        n194 = Get Date/Time In Seconds() -> (seconds since 1Jan1904=w246:timestamp)
        n195 = local read "total Points"() -> (w252:i32)
        n196 = Subtract(x=w246, y=w251) -> (x-y=w250:dbl)
        n197 = Subtract(x=w252, y=w249) -> (x-y=w247:i32)
        n198 = Divide(x=w249, y=w252) -> (x/y=w255:dbl)
        n199 = Divide(x=w250, y=w249) -> (x/y=w248:dbl)
        n200 = Multiply(x=w248, y=w247) -> (x*y=w245:dbl)
        "remaining" <- w245
        n201 = Multiply(x=w255, y=100.0) -> (x*y=→"Progress":dbl)
        n202 = Add(x=w246, y=w245) -> (x+y=→"ETA":timestamp)
      }
      frame "end" {
        n203 = Close File(refnum=w545) -> ()  [unwired: 1 in, 2 out]
        n204 = Unbundle By Name(w560) -> ("center X (m)"=w558:sgl, "center Y (m)"=w557:sgl, "angle (deg)"=w556:sgl, "width (m)"=w555:sgl, "height (m)"=w554:sgl)
        n205 = Bundle(w550, w550) -> (w572:cluster{sgl[][], sgl[][]})  [unwired: 1 in]
        n206 = Strip Path(path=w533) -> (stripped path=w541:path)  [unwired: 1 out]
        n207 = Close File(refnum=w543) -> (path=w542:path)  [unwired: 1 in, 1 out]
        n208 = local write "Status"("finishing" ("Status")) -> ()
        n209 = call "STSGrid.vi"("Binary Spectroscopy File"=w542) -> ()  [unwired: 11 in]
        n210 = Strip Path(path=w541) -> (stripped path=w540:path)  [unwired: 1 out]
        n211 = Build Array(w572) -> (w571:cluster{sgl[][], sgl[][]}[])
        n212 = Bundle By Name(cluster=T6 {"center X"=0.0, "center Y"=0.0, "angle"=0.0, "width"=0.0, "height"=0.0, "# pixels"=0, "# lines"=0} ("Scanfield"), "center X"=w558, "center Y"=w557, "angle"=w556, "width"=w555, "height"=w554, "# lines"=w551, "# pixels"=w552) -> (w553:T6)
        n213 = Path To String(path=w540) -> (string=w498:string)
        n214 = String To Path(string=w498) -> (path=w497:path)
        n215 = Strip Path(path=w533) -> (stripped path=w564:path, name=w563:string)
        n216 = Get Date/Time In Seconds() -> (seconds since 1Jan1904=w529:timestamp)
        n217 = Bundle By Name(cluster=T8 {"up/down"=FALSE, "time/line"=0.0, "start time"=timestamp(0 s since 1904-01-01), "end time"=timestamp(0 s since 1904-01-01)} ("Scan param"), "up/down"=TRUE, "time/line"=sgl nan ("input 7"), "start time"=w568, "end time"=w529) -> (w567:T8)
        n218 = Bundle("stripped path"=w564, "name"=w563) -> (w562:cluster{"stripped path":path, "name":string})  [unwired: 1 in]
        n219 = call <userlib>:"Save sxm File.vi"("Auto file naming? (T)"=FALSE, "Scanfield"=w553, "Scan param"=w567, "error in (no error)"=w561, "Channels data"=w571, "Channels config"=T7 [{"Name"="Z (m)", "Calibration"=1.0, "Offset"=0.0, "Channel index"=0}], "Filename control"=w562) -> ("error out"=w538:errorcluster)  [unwired: 2 in, 2 out]
        n220 = call <userlib>:"Get Session Path.vi"("error in (no error)"=w538, "Application ref in"=w537) -> ("error out"=w534:errorcluster, "Session path"=w536:path, "Application ref out"=w496:refnum<vi>)  [unwired: 7 in]
        n221 = call "SXM.vi"("Path"=w536, "Delete"=FALSE, "error in"=w534) -> ("error out"=w499:errorcluster)  [unwired: 7 in]
        n222 = Format Date/Time String(time format string (%c)=" Finished at %y%m%d - %H%M%S ", seconds (now)=w529) -> (date/time string=w528:string)  [unwired: 1 in]
        n223 = Path To String(path=w533) -> (string=w532:string)
        n224 = call <userlib>:"Set Session Path.vi"("Save settings to previous? (False)"=TRUE, "error in (no error)"=w499, "Session Folder"=w497, "Application ref in"=w496) -> ("error out"=w494:errorcluster, "Application ref out"=w495:refnum<vi>)  [unwired: 6 in]
        n225 = local read "zFile"() -> (w513:refnum<file>)
        n226 = Search and Replace String(input string="Email when finished", search string="@") -> (number of replacements=w524:i32)  [unwired: 6 in, 3 out]
        n227 = Concatenate Strings(w532, "\r\n", w528) -> (w531:string)
        n228 = call <userlib>:"BiasSpectroscopy SetProperties.vi"("Application ref in"=w495, "Z-Controller hold (no change)"=enum16{"no change", "on", "off"}."on") -> ("Application ref out"=w521:refnum<vi>)  [unwired: 12 in, 1 out]
        n229 = Close File(refnum=w513, error in=w494) -> (error out=w509:errorcluster)  [unwired: 1 out]
        n230 = Greater Than 0?(x=w524) -> (x > 0?=w523:bool)
        n231 = case shown="True" w523 {
          tunnel: w509 -> [w574 w579]
          tunnel: w531 -> [_ w577]
          tunnel: "Email when finished" -> [_ w576]
          tunnel: [w574 w575] -> w505
          frame False {
          }
          frame True {
            n232 = call "Send Email"("error in"=w579, "Message"=w577, "Subject"="Grid Finished", "Recipients"=w576) -> ("error out"=w575:errorcluster)  [unwired: 7 in]
          }
        }
        n233 = call <userlib>:"TipLift Set.vi"("TipLift (m)"=sgl 0.0, "Application ref in"=w521) -> ("Application ref out"=w518:refnum<vi>)  [unwired: 8 in, 1 out]
        n234 = call "move2mark (SubVI).vi"("Application in"=w518) -> ("Application out"=w504:refnum<vi>)  [unwired: 10 in]
        n235 = local read "Imaging Current"() -> (w502:dbl)
        n236 = call <userlib>:"Z-Ctrl Setpoint Set.vi"("Z Controller setpoint"=w502, "Application ref in"=w504) -> ("Application ref out"=w503:refnum<vi>)  [unwired: 8 in, 1 out]
        n237 = local read "Imaging Bias"() -> (w514:dbl)
        n238 = call "SafeBiasSet.vi"("Application ref in"=w503, "Bias (V)"=w514, "error in (no error)"=w505) -> ("Application ref out"=w515:refnum<vi>, "Error out"=w508:errorcluster)  [unwired: 6 in]
        n239 = call <userlib>:"Ctrl-on_off Set.vi"("error in (no error)"=w508, "Z Controller ON/OFF"=TRUE, "Application ref in"=w515) -> ("error out"=w507:errorcluster, "Application ref out"=w517:refnum<vi>)  [unwired: 7 in]
        n240 = call <userlib>:"Point Erase.vi"("Application ref in"=w517, "Point index (-1=All points)"=0, "error in (no error)"=w507) -> ("Application ref out"=w511:refnum<vi>, "error out"=w506:errorcluster)  [unwired: 11 in]
        n241 = call "PLL_On_Off (SubVI).vi"("error in (no error)"=w506, "Output ON/OFF (F=OFF)"=FALSE, "Application in"=w511) -> ("error out"=w501:errorcluster, "Application out"=w512:refnum<vi>)  [unwired: 7 in]
      }
    }
    "Error out" <- w36
    "Points taken" <- w10
    "X Offset" <- w9
    "Y Offset" <- w8
  }
